vi "Read set period.vi"(8 "error in":errorcluster, 11 "timing source in":refnum<class "scan engine timing source.lvclass">) -> (0 "error out":errorcluster, 2 "set period":bool, 3 "timing source out":refnum<class "scan engine timing source.lvclass">)   [LabVIEW 2013, in "scan engine timing source.lvclass"]
doc: "Indicates whether or not the <b>set period</b> flag is set in the object. If it is, initialize will set the period of the scan engine. If false, the period will not be set."
uses:
  scan engine timing source.lvclass
  scan engine timing source.lvclass/scan engine timing source.ctl
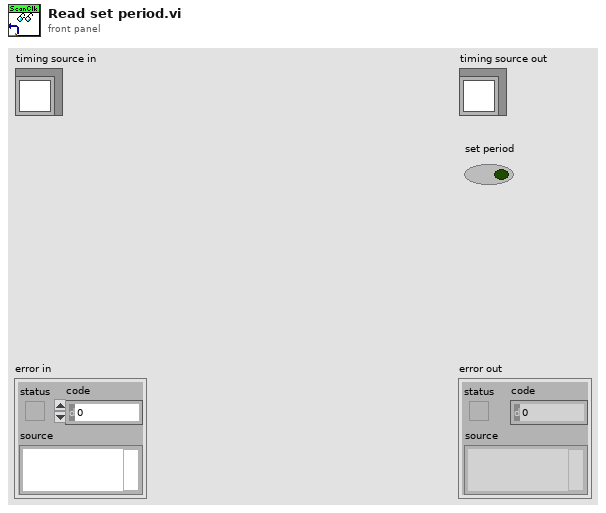
[diagram p1: front panel]
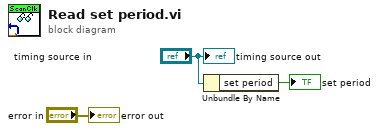
[diagram p0: block diagram]
diagram:
  n1 = Unbundle By Name("timing source in") -> ("set period"=→"set period":bool)
  "error out" <- "error in"
  "timing source out" <- "timing source in"
